vi "Pins to NI-AWG Sessions.vi"(8 "error in (no error)":errorcluster, 9 "Pins":string[](array[string]), 10 "Semiconductor Module Context":T1) -> (0 "error out":errorcluster, 1 "Channel Lists":string[](array[string]), 2 "Semiconductor Module Context Out":T1, 3 "Instrument Sessions":refnum<k15>[](array[refnum]))   [LabVIEW 2013]
uses:
  <vilib>/NI_TestStand_SemiconductorModule/NI_TestStand_Semiconductor_Module.lvlibp/PinMap/General/SemiconductorModuleContext.ctl
  <vilib>/NI_TestStand_SemiconductorModule/NI_TestStand_Semiconductor_Module.lvlibp
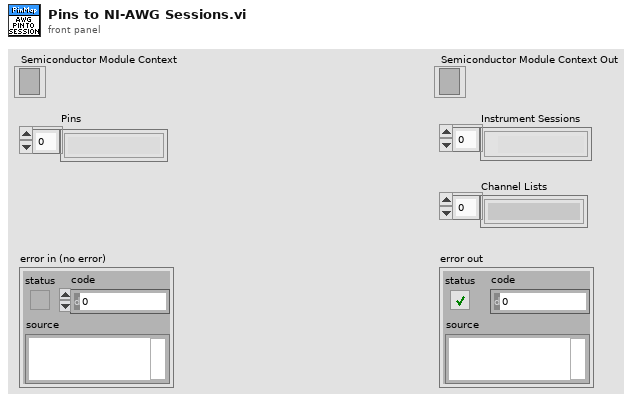
[diagram p1: front panel]
types:
  T1 = typedef "NI_TestStand_Semiconductor_Module.lvlibp/SemiconductorModuleContext.ctl" = refnum<k7>
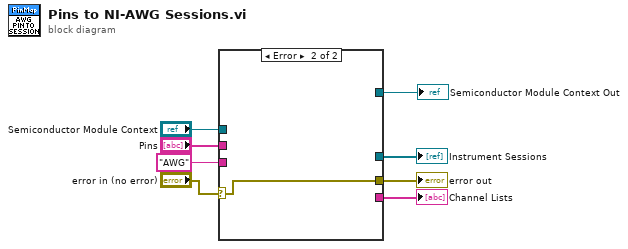
[diagram p0: block diagram]
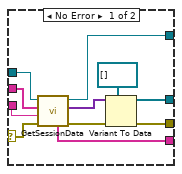
[diagram p2: hidden frame]
diagram:
  n1 = case shown="Error" "error in (no error)" {
    selector: "error in (no error)" -> [w9 w20]
    tunnel: "Semiconductor Module Context" -> [w19 _]
    tunnel: "Pins" -> [w18 _]
    tunnel: "AWG" ("Instrument Type Id") -> [w17 _]
    tunnel: [w16 _] -> w5
    tunnel: [w13 _] -> w4
    tunnel: [w11 _] -> w3
    tunnel: [w10 w20] -> w2
    frame No Error {
      n2 = call <vilib>:"GetSessionData.vi"("error in (no error)"=w9, "Instrument Type Id"=w17, "Pins"=w18, "Semiconductor Module Context"=w19) -> ("error out"=w15:errorcluster, "Session Data"=w14:variant[], "Semiconductor Module Context Out"=w13:T1, "Channel Lists"=w16:string[])  [unwired: 2 in, 2 out]
      n3 = Variant To Data(error in=w15, type=refnum<k15>[] [], Variant=w14) -> (data=w11:refnum<k15>[], error out=w10:errorcluster)
    }
    frame Error {
    }
  }
  "Channel Lists" <- w5
  "Semiconductor Module Context Out" <- w4
  "Instrument Sessions" <- w3
  "error out" <- w2
